vi "Get Current Time if Not Set.vi"(11 "Start Time":timestamp) -> (3 "seconds since 1Jan1904":timestamp)   [LabVIEW 2020, in "Thermal Chamber Response Simlator.lvclass"]
uses:
  Thermal Chamber Response Simlator.lvclass
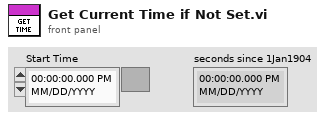
[diagram p1: front panel]
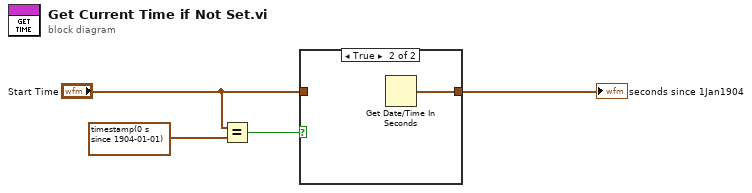
[diagram p0: block diagram]
diagram:
  n1 = Equal?(x="Start Time", y=timestamp(0 s since 1904-01-01) ("Start Time")) -> (x = y?=w2:bool)
  n2 = case shown="True" w2 {
    tunnel: [w5 w6] -> w3
    tunnel: "Start Time" -> [w5 _]
    frame False {
    }
    frame True {
      n3 = Get Date/Time In Seconds() -> (seconds since 1Jan1904=w6:timestamp)
    }
  }
  "seconds since 1Jan1904" <- w3
